vi "rethinkdb_handshake_final.vi"(8 "error in (no error)":errorcluster, 9 "client_first_message":string, 10 "password":string, 11 "server_response (json)":string="{\"success\":true,\"min_protocol_version\":0,\"max_protocol_version\":0,\"server_version\":\"2.3.0\"}\u0000\n{\"success\":true,\"authentication\":\"r=rOprNGfwEbeRWgbNEkqO%hvYDpWUa2RaTCAfuxFIlj)hNlF$k0,s=W22ZaJ0SNY7soEsUEjb6gQ==,i=4096\"}\u0000") -> (0 "error out":errorcluster, 3 "authentication_request":string)   [LabVIEW 2017]
uses:
  b02b9132-5309-4610-a6c0-a0c94150cd68.vi
  dab8a8d9-9bd0-4e10-b8f7-9264eab402ee.vi
  json/json_resolve_key.vi
panel:
  out "success?":bool
  out "server_first_message":string
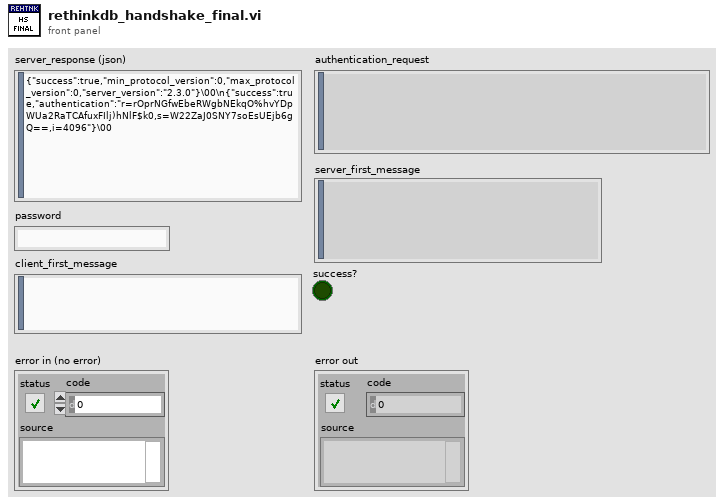
[diagram p1: front panel]
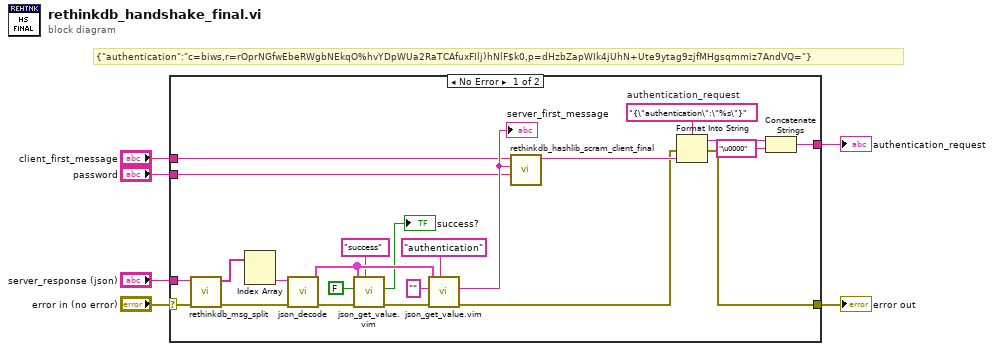
[diagram p0: block diagram]
diagram:
  # "{\"authentication\":\"c=biws,r=rOprNGfwEbeRWgbNEkqO%hvYDpWUa2RaTCAfuxFIlj)hNlF$k0,p=dHzbZapWIk4jUhN+Ute9ytag9zjfMHgsqmmiz7AndVQ=\"}"
  n1 = case shown="No Error" "error in (no error)" {
    selector: "error in (no error)" -> [w29 w30]
    tunnel: [w27 w30] -> w5
    tunnel: [w26 _] -> w4
    tunnel: "server_response (json)" -> [w28 _]
    tunnel: "client_first_message" -> [w8 _]
    tunnel: "password" -> [w7 _]
    frame No Error {
      w24 = "{\"authentication\":\"%s\"}"  # authentication_request
      n2 = call "rethinkdb_msg_split.vi"("error in (no error)"=w29, "data in"=w28) -> ("error out"=w16:errorcluster, "messages"=w25:string[])  [unwired: 7 in, 1 out]
      n3 = Index Array(array=w25) -> (element #2=w21:string)  [unwired: 2 in, 1 out]
      n4 = call "json_decode.vi"("error in (no error)"=w16, "json"=w21) -> ("error out"=w20:errorcluster, "pairs"=w18:cluster{"key":string, "value":variant}[])  [unwired: 8 in]
      n5 = call "json_get_value.vim"("key"="success", "error in (no error)"=w20, "default"=FALSE, "pairs"=w18) -> ("error out"=w19:errorcluster, "value"=→"success?":bool)  [unwired: 5 in, 1 out]
      n6 = call "json_get_value.vim"("key"="authentication", "error in (no error)"=w19, "default"="", "pairs"=w18) -> ("error out"=w10:errorcluster, "value"=w9:string)  [unwired: 5 in, 1 out]
      "server_first_message" <- w9
      n7 = call "rethinkdb_hashlib_scram_client_final.vi"("password"=w7, "server_first_message"=w9, "client_first_message"=w8) -> ("client_final_message"=w11:string)  [unwired: 8 in]
      n8 = Format Into String(format string=w24, error in=w10, w11) -> (resulting string=w23:string, error out=w27:errorcluster)  [unwired: 1 in]
      n9 = Concatenate Strings(w23, "\u0000" ("string")) -> (w26:string)
    }
    frame Error {
    }
  }
  "error out" <- w5
  "authentication_request" <- w4
